vi "decipher_incoming_lineitem.vi"(2 "lineitem (in)":string, 5 "error in (no error)":errorcluster) -> (15 "lineitem_type (out)":T1=enum."received.dostep", 16 "clustered_item (out)":T2, 17 "timestep (out)":dbl, 19 "error out":errorcluster)   [LabVIEW 2016]
uses:
  controls/entity.ctl
  controls/entity_type.ctl
  controls/lineitem_types.ctl
  controls/group.ctl
panel:
  in  "lineitem_options (hidden)":T1=enum."received.dostep"
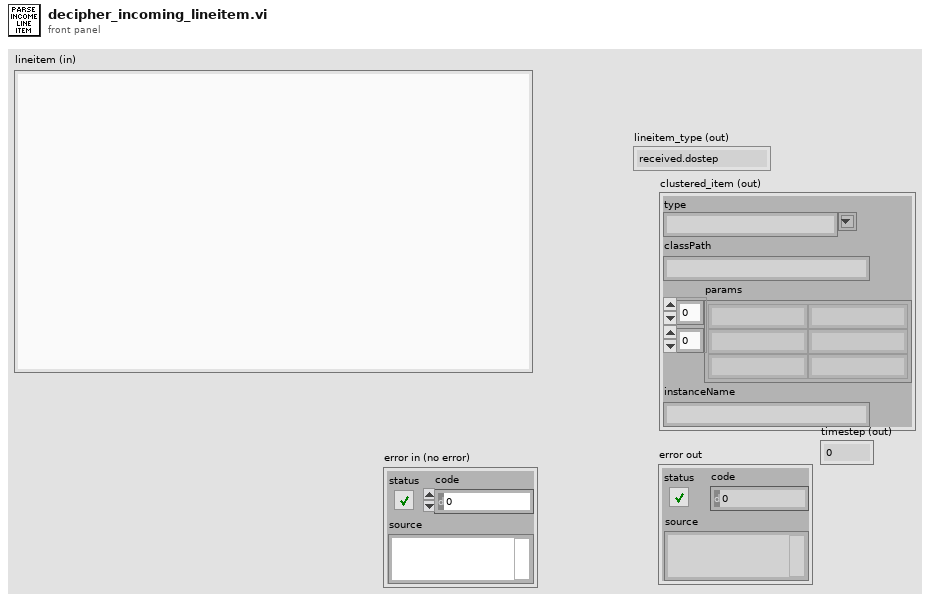
[diagram p1: front panel]
types:
  T1 = typedef "lineitem_types.ctl" = enum16{"<unknown>", "received.dostep", "received.item", "received.simend"}
  T2 = typedef "entity.ctl" = cluster{"type":T3, "classPath":string, "params":string[][], "instanceName":string}
  T3 = typedef "entity_type.ctl" = string
  T4 = typedef "group.ctl" = cluster{"timeStep":dbl, "entities":T2[]}
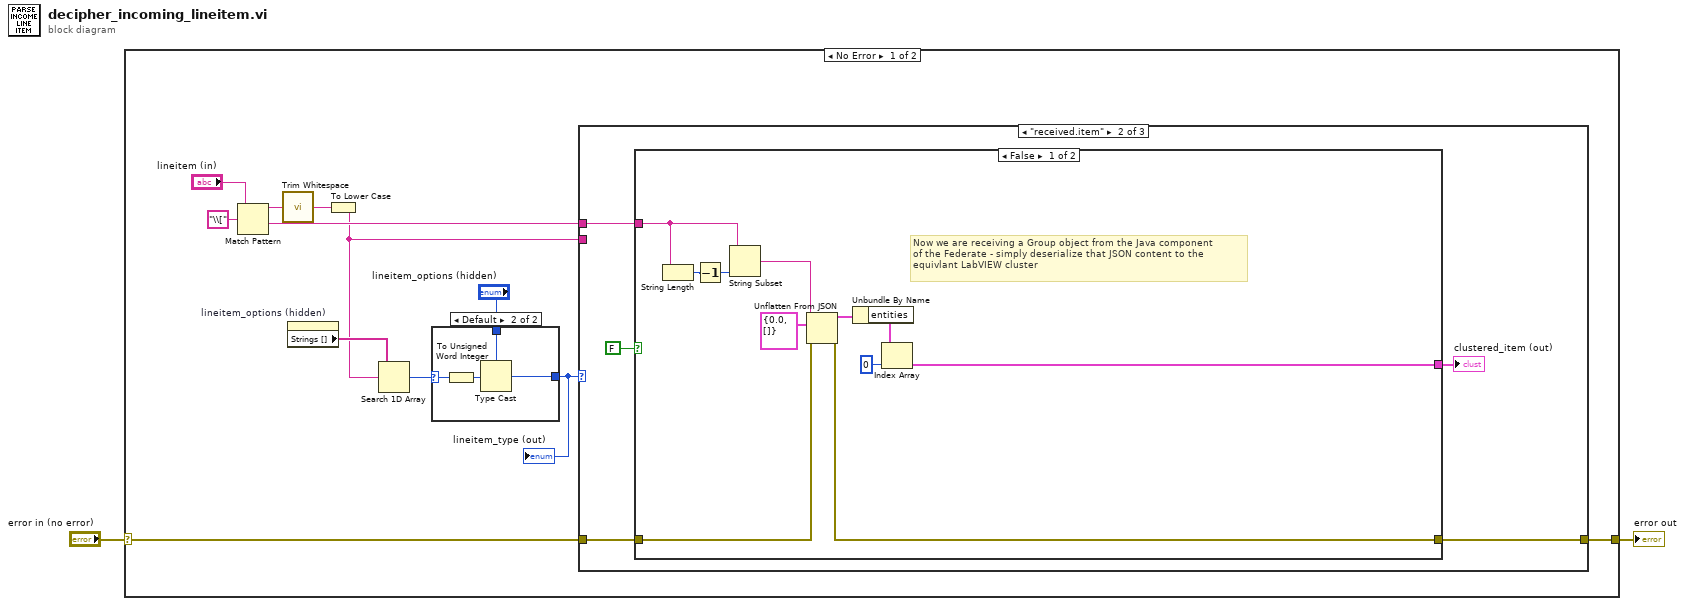
[diagram p0: block diagram]
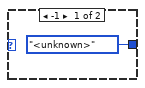
[diagram p2: hidden frame]
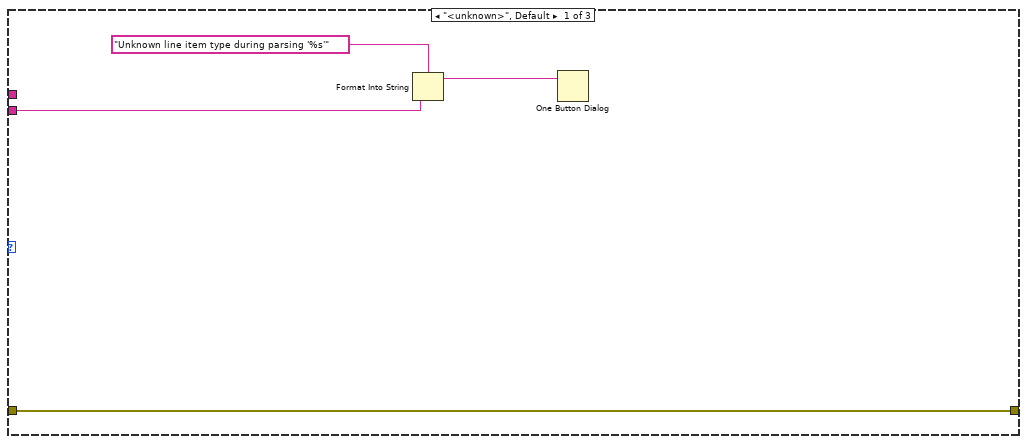
[diagram p3: hidden frame]
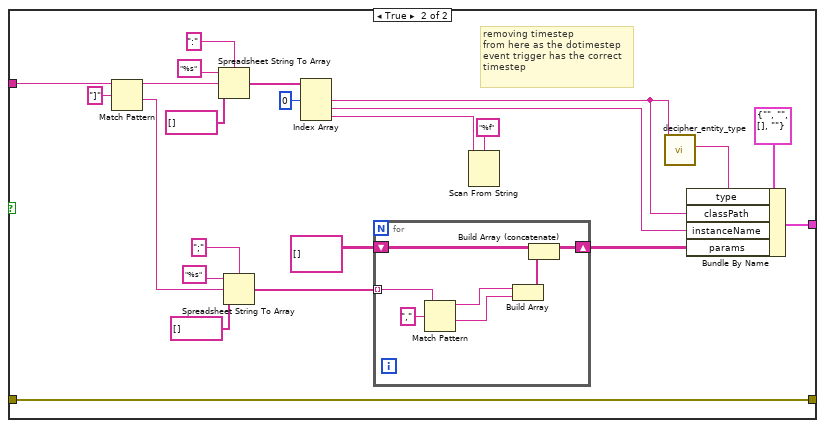
[diagram p4: hidden frame]
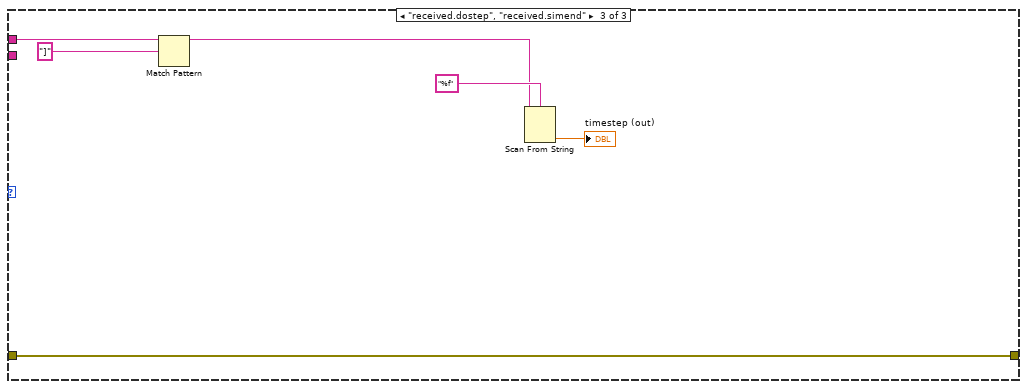
[diagram p5: hidden frame]
diagram:
  n1 = case shown="No Error" "error in (no error)" {
    selector: "error in (no error)" -> [w6 w76]
    tunnel: [w5 w76] -> w1
    frame No Error {
      n2 = Match Pattern(string="lineitem (in)", regular expression="\\[") -> (before substring=w13:string, after substring=w12:string)  [unwired: 1 in, 2 out]
      n3 = call <vilib>:"Trim Whitespace.vi"("string"=w13) -> ("trimmed string"=w10:string)  [unwired: 1 in]
      n4 = property on="lineitem_options (hidden)" class="Enum (strict)"() -> ("Strings []"=w9:string[])  [unwired: 2 in, 2 out]
      n5 = To Lower Case(string=w10) -> (all lower case string=w3:string)
      n6 = Search 1D Array(1D array=w9, element=w3) -> (index of element=w7:i32)  [unwired: 1 in]
      n7 = case shown="Default" w7 {
        selector: w7 -> [_ w16]
        tunnel: "lineitem_options (hidden)" -> [_ w19]
        tunnel: [lineitem_types."<unknown>" ("lineitem_options (hidden)") w18] -> w4
        frame -1 {
        }
        frame Default {
          n8 = To Unsigned Word Integer(number=w16) -> (unsigned 16bit integer=w17:u16)
          n9 = Type Cast(type=w19, x=w17) -> (*(type *) &x=w18:T1)
        }
      }
      "lineitem_type (out)" <- w4
      n10 = case shown="\"received.item\"" w4 {
        tunnel: w12 -> [_ w24 w72]
        tunnel: w6 -> [w23 w27 w71]
        tunnel: [w23 w25 w71] -> w5
        tunnel: w3 -> [w21 _ _]
        frame "<unknown>", Default {
          n11 = Format Into String(format string="Unknown line item type during parsing '%s'", w21) -> (resulting string=w20:string)  [unwired: 2 in, 1 out]
          n12 = One Button Dialog(message=w20) -> ()  [unwired: 1 in, 1 out]
        }
        frame "received.item" {
          n13 = case shown="False" FALSE {
            tunnel: [w35 w56] -> w28
            tunnel: w27 -> [w34 w44]
            tunnel: w24 -> [w30 w40]
            tunnel: [w33 w44] -> w25
            frame False {
              # "Now we are receiving a Group object from the Java component\nof the Federate - simply deserialize that JSON content to the\nequivlant LabVIEW cluster"
              n14 = String Length(string=w30) -> (length=w32:i32)
              n15 = Decrement(x=w32) -> (x-1=w31:i32)
              n16 = String Subset(string=w30, length (rest)=w31) -> (substring=w29:string)  [unwired: 1 in]
              n17 = Unflatten From JSON(JSON string=w29, type and defaults=T4 {"timeStep"=0.0, "entities"=[]} ("group"), error in (no error)=w34) -> (value=w38:T4, error out=w33:errorcluster)  [unwired: 4 in]
              n18 = Unbundle By Name(w38) -> ("entities"=w37:T2[])
              n19 = Index Array(array=w37, index=0) -> (element=w35:T2)
            }
            frame True {
              # "removing timestep\nfrom here as the dotimestep\nevent trigger has the correct\ntimestep"
              n20 = Match Pattern(string=w40, regular expression="]") -> (before substring=w41:string, after substring=w42:string)  [unwired: 1 in, 2 out]
              n21 = Spreadsheet String To Array(delimiter (Tab)=":", format string="%s", spreadsheet string=w41, array type (2D Dbl)=string[] []) -> (array=w51:string[])
              n22 = Spreadsheet String To Array(delimiter (Tab)=";", format string="%s", spreadsheet string=w42, array type (2D Dbl)=string[] []) -> (array=w57:string[])
              n23 = Index Array(array=w51, index #1=0 ("index")) -> (element #1=w46:string, element #2=w49:string, element #3=w48:string)  [unwired: 2 in]
              n24 = for {
                tunnel: w57 -> [w68] mode=indexing
                shift-right: [w63] -> w47
                shift-left: string[][] [] -> [w65]
                n25 = Match Pattern(string=w68, regular expression=",") -> (before substring=w67:string, after substring=w66:string)  [unwired: 1 in, 2 out]
                n26 = Build Array(w67, w66) -> (w64:string[])
                n27 = Build Array (concatenate)(w65, w64) -> (w63:string[][])
              }
              n28 = Scan From String(format string="%f", input string=w48) -> ()  [unwired: 4 in, 3 out]
              n29 = call "decipher_entity_type.vi"("classpath (fully qualified)"=w46) -> ("entity_type (out)"=w45:T3)  [unwired: 10 in]
              n30 = Bundle By Name(cluster=T2 {"type"="", "classPath"="", "params"=[], "instanceName"=""} ("entity"), "type"=w45, "classPath"=w46, "instanceName"=w49, "params"=w47) -> (w56:T2)
            }
          }
          "clustered_item (out)" <- w28
        }
        frame "received.dostep", "received.simend" {
          n31 = Match Pattern(string=w72, regular expression="]") -> (before substring=w70:string)  [unwired: 1 in, 3 out]
          n32 = Scan From String(format string="%f", input string=w70) -> (output 1=→"timestep (out)":dbl)  [unwired: 3 in, 3 out]
        }
      }
    }
    frame Error {
    }
  }
  "error out" <- w1
